vi "HFRR ADV v033 new software.vi"() -> ()   [LabVIEW 2025] (continued)
  # "System Control Commands\nS;1 - Starts the full automation cycle (Runs Priming-humidify till 70RH sequence first, then switches to Maintenance).\nS;0 - Stops the system immediately and enters Standby mode (Safe State: All actuators OFF).\nM;1 - Skips the priming sequence and jumps directly to Maintenance mode (PID control).\nR;1 - Resets the logic state machine and clears all errors, returning to Standby.\nService Mode (Manual Control)\nX;1 - Enters Manual Service Mode. This disables all automatic logic, sensor safety checks, and timers.\nX;0 - Exits Manual Service Mode and returns to Standby (Safe State).\nActuator Commands (Only work after sending X;1)\nP;[0-255] - Sets the Pump PWM. Note that this is Active Low (0 = Max Flow, 255 = Pump OFF).\nF;I;[0-255] - Sets the Intake Fan speed (0 = OFF, 255 = Max Speed).\nF;O;[0-255] - Sets the Exhaust Fan speed (0 = OFF, 255 = Max Speed).\nD;1 - Turns the Dehumidifier Relay ON.\nD;0 - Turns the Dehumidifier Relay OFF."
  # "%RH"
  # "ISO : WS1.4"
  # "Start test and end test log--- done\nDisable heater ON and Humidity ON during the test --- done\ntemprature and ---done\nhumidity reach log\nauto start run true logic and log\nmanual start log once"
  # "Reference Fluid Information"
  # "Note:\nMake sure to place all images in the folder \"C:\\WinDucom\\im\" before clicking on \"Import Image.\""
  # "NOTE:\nPlace all the images in the path \"C:\\WinDucom\\im\" before clicking on Import Image"
  # "Wear Scar Measurements"
  # "Reference Fluid Information"
  # "Graph :"
types:
  T1 = enum32{"Home", "Dashboard", "Imaging", "Report", "Analysis", "About", "Test Setup", "Advance", "Calibration"}
  T2 = enum32{"HOME", "Test Setup", "Acquire", "Adv Scar", "Adv Scar Report", "Compare Files", "Calibration", "About", "Advance", "Mooha"}
  T3 = enum16{"ASTM D6079", "ISO 12156", "CEC F-096-A-06", "Custom"}
  T4 = enum32{"Dashboard 1", "Dashboard 2", "Dashboard 3"}
  T5 = enum32{"COF", "Friction", "ECR", "Temperature", "Humidity", "Stroke"}
  T6 = enum32{"Coefficient Of Friction", "Air Temperature", "Humidity", "Stroke", "Sample Temperature", "Electrical Contact Resistance", "Frequency", "Air Temp vs Rh"}
  T7 = enum32{"Main", "Stroke", "Friction", "Temperature"}
  T8 = enum32{"Stroke Calibration", "Friction Force Calibration", "Temperature Calibration", "Default"}
  T9 = enum32{"Step 1", "Step 2", "Step 3", "Step 4", "Step 5", "Step 6", "Step 7", "Step 8", "Step 9"}
  T10 = enum32{"Test Progress", "Stroke Points Completed"}
  T11 = enum32{"Page 1", "Page 2", "Page 3", "Page 4", "Page 5", "Page 6"}
  T12 = enum32{"Main", "Step 1", "Step 2", "Step 3", "Air Step 1", "Air Step 2", "Air Step 3"}
  T13 = enum32{"Air Temperature", "Sample Temperature", "Default"}
  T14 = enum32{"COMMUNICATION", "CALIBRATION", "Temp Variables", "Camera", "WO 2465 (1)", "WO 2465 (2)", "WO 2465 (3)"}
  T15 = typedef "Auto Start enum.ctl" = enum16{"Init", "Humidity & Temperature On", "Reach point", "Maintain Stage", "Start Stage", "close", "Exit"}
  T16 = typedef "imagedata.ctl" = cluster{"image type":i32, "image depth":i32, "image":u8[], "mask":u8[], "colors":u32[], "Rectangle":cluster{"left":i16, "top":i16, "right":i16, "bottom":i16}}
  T17 = enum32{"HOME", "Test Setup", "Acquire", "Compare Files", "Print Report", "About", "Advance", "Mooha"}
  T18 = cluster{"Read Heave and Surge":string, "Bytes at Heave Port":dbl, "Heave and Surge COM Port:":refnum<visa-resource-name>, "Com Port 2":refnum<visa-resource-name>, "Residual Due":string, "Heave COM Status 2":bool, "Heave COM Status":bool, "Port 2":bool, "Sway PPR":dbl, "Surge PPR":dbl, "Heave PPR":dbl, "Sway Pitch":dbl, "Surge Pitch":dbl, "Heave Pitch":dbl, "Sway Pulses/mm":dbl, "Surge Pulses/mm":dbl, "Heave Pulses/mm":dbl, "inner loop":dbl, "Read Heave and Surge 2":string, "String 36":string, "Write S":bool, "WriteCC1":string[], "Heave COM Loop":i32, "LastCom":string, "EXIT":bool, "Error Heave":errorcluster}
  T19 = enum8{"Enabled", "Disabled", "Disabled and Grayed Out"}
  T20 = cluster{"Read Uno":string, "Bytes at Heave Port":dbl, "UNO COM Port:":refnum<visa-resource-name>, "UNO COM Port: 2":refnum<visa-resource-name>, "Residual Due":string, "UNO COM Status 2":bool, "UNO COM Status":bool, "Port 2":bool, "Sway PPR":dbl, "Surge PPR":dbl, "Heave PPR":dbl, "Sway Pitch":dbl, "Surge Pitch":dbl, "Heave Pitch":dbl, "Sway Pulses/mm":dbl, "Surge Pulses/mm":dbl, "Heave Pulses/mm":dbl, "inner loop":dbl, "Read Heave and Surge 2":string, "String 36":string, "Write S":bool, "WriteCC1":string[], "Heave COM Loop":i32, "LastCom":string, "EXIT":bool, "Error Heave":errorcluster}
  T21 = enum32{"HOME", "Test Setup", "Acquire", "Adv Scar", "Adv Scar Report", "Compare Files", "About", "Advance", "Mooha"}
  T22 = typedef "POST ANALYSIS ENUM.ctl" = enum16{"OPEN EXE", "INIT", "OPEN FILE", "FIT", "DRAW REC", "DRAW LINE", "PAN", "ZOOM IN", "ZOOM OUT", "SET ZOOM", "CLEAR ROI", "GET MEASUREMENTS", "RESIZE MODE", "STREAM START", "STREAM STOP", "SHOW UI", "MINIMIZE UI", "HIDE UI", "CKISE APP", "CLOSE CONNECTION", "SAVE IMAGE", "SET ROI COLOR", "READ", "TCP CHECK", "CLOSE"}
  T23 = typedef "CAMERA LIVE FEED ENUM.ctl" = enum16{"OPEN EXE", "INIT", "READ", "CAMERA CONNECT", "CAMERA START", "CAMERA STOP", "CAMERA GRAY", "CAMERA RGB", "CAMERA MINIMIZE", "CAMERA CLOSE", "CAMERA MODE LIST", "CAMERA MODE SET", "CAMERA RESTORE", "CAMERA SAVE", "CLOSE"}
  T24 = enum16{"Always On", "Always Off", "Off While Running"}
  T25 = enum32{"Home", "Dashboard", "Imaging", "Report", "Analysis", "About", "Test Setup", "Advance"}
  T26 = cluster{"File Name":string, "Test Method":string, "Operator":string, "Fuel Description":string, "Date and time":string}
  T27 = enum32{"Home", "Dashboard", "Imaging", "Report", "Analysis", "About", "Test Setup"}
  T28 = enum32{"HOME", "Test Setup", "Acquire", "Compare Files", "About", "Advance", "Mooha"}
  T29 = typedef "NI_ReportGenerationCore.lvlib/HTML Report Image Alignment.ctl" = enum16{"(default)", "LEFT", "RIGHT", "TOP", "TEXTTOP", "MIDDLE", "ABSMIDDLE", "BASELINE", "BOTTOM", "ABSBOTTOM"}
  T30 = cluster{"y":dbl, "LVDT STROKE DISPLAY":dbl, "y":dbl}
  T31 = enum16{"INIT", "READ", "MANUAL WRITE", "WRITE", "CLOSE", "ERROR INIT"}
diagram:
  w3 = 0.0 ("ch0_filt")
  w5 = -9999999.0 ("max_ch0")
  w6 = 9999999.0 ("min_ch0")
  w17 = FALSE ("Visible")
  w18 = T19."Enabled" ("Disabled")
  w21 = FALSE ("Visible")
  w20 = FALSE ("Humidity Off Command")
  w36 = "" ("USER ID")
  (unwired) T21."HOME" ("Main Tab")
  # "[CH1]    - FF\n[CH2]   - TEMPERATURE\n[CH3]    - Humidity\n[CH4]    - AIR TEMP\n[CH5]\\- Visa Uno\n[CH6] \\- Visa Due\n[CH7]  \\- file path\n[CH8]   - Displacement Gain\n[CHA]   - Stroke Gain\n[CHB]   - Stroke PID Gain\n[CHC]   -Language Selection\n[CHD]   -Power +\n[CHE]   -Power_\n[CHF]   -Heater\n[CHG]   -Humidity Wet\n[CHH]   -Humidity Dry\n[CHI]   -Integral Time \n[CHIJ   -Air intercept\n[CHI]   -Temp Intercept"
  n1 = local write "Cal Password"("" ("Cal Password")) -> ()
  n2 = property on="Auto Start Test" class="Bool (strict)"("Visible"=TRUE) -> ()  [unwired: 2 in, 2 out]
  n3 = property on="FRICVALZ 2" class="Bool (strict)"("DisabledEnum"=w18) -> ()  [unwired: 2 in, 2 out]
  n4 = property on="FRICVALZ 4" class="Bool (strict)"("DisabledEnum"=w18) -> ()  [unwired: 2 in, 2 out]
  n5 = property on="FRICVALZ 3" class="Bool (strict)"("DisabledEnum"=w18) -> ()  [unwired: 2 in, 2 out]
  n6 = property on="About" class="Clust (strict)"("Visible"=FALSE) -> ()  [unwired: 2 in, 2 out]
  n7 = property on="Wrong Password" class="Str"("Visible"=w17) -> ()  [unwired: 2 in, 2 out]
  n8 = property on="Calibration 2" class="TabCtl (strict)"("Visible"=w17) -> ()  [unwired: 2 in, 2 out]
  n9 = flat-sequence {
    tunnel: [w57] -> w2
    tunnel: [w102] -> w28
    tunnel: w2 -> [w97]
    tunnel: [w103] -> w30
    tunnel: w28 -> [w103]
    tunnel: w30 -> [w163]
    tunnel: [w163] -> w29
    tunnel: w29 -> [w194]
    tunnel: [w194] -> w39
    tunnel: w39 -> [w201]
    tunnel: [w207] -> w27
    tunnel: [w195] -> w26
    tunnel: [w249] -> w1
    tunnel: [w248] -> _
    tunnel: w27 -> [w248]
    tunnel: w26 -> [w249]
    frame #0 {
      n10 = call "CLOSE CONNECTION.vi"("error in (no error)"="error in (no error) 2") -> ("error out"=w62:errorcluster)  [unwired: 10 in]
      n11 = call <vilib>:"Clear Errors.vi"("error in (no error)"=w62) -> ("error out"=w61:errorcluster)  [unwired: 5 in, 1 out]
      n12 = disable-structure shown="Enabled" {
        disable-tunnel: w61 -> [w89 _]
        disable-tunnel: [w88 _] -> w60
        frame Enabled {
          n13 = call <userlib>:"Fit VI window to Largest Dec.vi"("error in (no error)"=w89, "border spacing (2 px)"=1) -> ("error out"=w92:errorcluster, "dup VI Ref"=w96:refnum<vi>)  [unwired: 4 in]
          n14 = invoke on="Invoke Node" class="VI" method="FP.Run-Time Position.Maximized"(reference=w96, error in=w92) -> (error out=w93:errorcluster)  [unwired: 2 in, 3 out]
          n15 = call <vilib>:"Clear Errors.vi"("error in (no error)"=w93) -> ("error out"=w95:errorcluster)  [unwired: 5 in, 1 out]
          n16 = control-ref of="This VI"() -> (w87:refnum<vi>)
          n17 = invoke on="Invoke Node" class="VI" method="Default Vals.Reinit All"(reference=w87, error in=w95) -> (reference out=w91:refnum<vi>, error out=w90:errorcluster)  [unwired: 1 in, 1 out]
          n18 = Close Reference(reference=w91, error in (no error)=w90) -> (error out=w88:errorcluster)
        }
        frame Disabled {
        }
      }
      n19 = call "Stall Data Flow.vim"("value in"=w60, "milliseconds to wait"=u32 2000) -> ("value out"=w59:errorcluster)  [unwired: 1 out]
      n20 = call "Read Config.vi"("error in (no error)"=w59) -> ("error out"=w57:errorcluster, "STROKE PARAMETERS"=w68:dbl[], "ADC PARAMETERS"=w69:dbl[], "PID  PARAMETERS"=w70:dbl[], "Stroke Calibration"=w67:string)  [unwired: 6 in]
      n21 = Index Array(array=w68) -> (element #1=w85:dbl, element #2=w86:dbl)  [unwired: 2 in]
      n22 = Index Array(array=w69) -> (element #1=w81:dbl, element #2=w82:dbl, element #3=w83:dbl, element #4=w84:dbl)  [unwired: 4 in]
      n23 = Index Array(array=w70) -> (element #1=w72:dbl, element #2=w73:dbl, element #3=w74:dbl, element #4=w75:dbl, element #5=w76:dbl, element #6=w77:dbl, element #7=w78:dbl, element #8=w79:dbl, element #9=w80:dbl)  [unwired: 9 in]
      n24 = local write "milliseconds to wait"(w72) -> ()
      n25 = local write "dt"(w73) -> ()
      n26 = local write "kp"(w74) -> ()
      n27 = local write "ki"(w75) -> ()
      n28 = local write "kd"(w76) -> ()
      n29 = local write "max_step_change"(w77) -> ()
      n30 = local write "max_amplitude"(w78) -> ()
      n31 = local write "min_amplitude"(w79) -> ()
      n32 = local write "startup_cmd"(w80) -> ()
      n33 = local write "VREF"(w81) -> ()
      n34 = local write "ADC_Resolution"(w82) -> ()
      n35 = local write "PIEZO_CAL_FACTOR"(w83) -> ()
      n36 = local write "NORMAL_FORCE"(w84) -> ()
      n37 = local write "STROKE FILTER"(w85) -> ()
      n38 = local write "Add up Stroke"(w86) -> ()
      n39 = Spreadsheet String To Array(delimiter (Tab)=";", format string="", spreadsheet string=w67, array type (2D Dbl)=dbl[] []) -> (array=w71:dbl[])
      n40 = local write "calibration values"(w71) -> ()
    }
    frame #1 {
      n41 = property on="Auto Scar Check" class="Clust (strict)"("Visible"=TRUE) -> ()  [unwired: 2 in, 2 out]
      n42 = property on="Sign In" class="Bool (strict)"("DisabledEnum"=T19."Disabled" ("Disabled")) -> ()  [unwired: 2 in, 2 out]
      n43 = local write "sign in temp"(FALSE ("sign in temp")) -> ()
      n44 = call "dialog box.vi"("Status"="Before starting the test, verify that the microscope cable is connected.", "error in"=w97) -> ("error out"=w102:errorcluster)  [unwired: 8 in]
    }
    frame #2 {
      (unwired) TRUE ("Re-Initialise")
      # "kkkkk"
      # "C:\\Windows\\wndcm_pw_stdED hfrr.txt"
      # "C:\\LAB-IQ NXT"
      # "C:\\LAB-IQ NXT\\wndcm_pw_stdED hfrr.txt"
      # "password file"
      n45 = Current VI's Path() -> (path=w119:path)
      n46 = Strip Path(path=w119) -> (stripped path=w112:path)  [unwired: 1 out]
      n47 = local write "main tab sub"(enum32{"Page 1", "Page 2"}."Page 1" ("main tab sub")) -> ()
      n48 = local write "Main Tab Display"(T4."Dashboard 1" ("Main Tab Display")) -> ()
      n49 = local write "Main Tab"(T2."HOME" ("Main Tab")) -> ()
      n50 = Path To String(path=w112) -> (string=w114:string)
      n51 = Search/Split String(string=w114, search string/char (-)=".exe") -> (match + rest of string=w116:string)  [unwired: 1 in, 2 out]
      n52 = Match True/False String(2:".vi" ("false string"), 3:".exe" ("true string"), 4:w116) -> (0:w113:bool)  [unwired: 1 out]
      n53 = List Folder(path=path "C:/LAB-IQ" ("directory path"), pattern="*.txt") -> (filenames=w125:string[])  [unwired: 2 in, 3 out]
      n54 = case shown="True" w113 {
        tunnel: w112 -> [w134 w136]
        tunnel: [w134 w135] -> w110
        frame False {
        }
        frame True {
          n55 = Strip Path(path=w136) -> (stripped path=w135:path)  [unwired: 1 out]
        }
      }
      n56 = Search 1D Array(1D array=w125, element="wndcm_pw_stdED hfrr.txt") -> (index of element=w128:i32)  [unwired: 1 in]
      n57 = Equal?(x=w128, y=-1) -> (x = y?=w123:bool)
      n58 = Path To String(path=w110) -> (string=→"Gain path":string)
      n59 = case shown="True" w123 {
        frame False {
        }
        frame True {
          n60 = String To Byte Array(string="123\n") -> (unsigned byte array=w141:u8[])
          n61 = Array Size(array=w141) -> (size(s)=w140:i32)
          n62 = for {
            N: w140 -> [_]
            tunnel: w141 -> [w154]
            tunnel: [w151] -> w143 mode=indexing
            tunnel: w140 -> [w146]
            i -> [w144]
            n63 = Decrement(x=w146) -> (x-1=w147:i32)
            n64 = Index Array(array=w154, index=w144) -> (element=w153:u8)
            n65 = Equal?(x=w144, y=w147) -> (x = y?=w148:bool)
            n66 = Number To Decimal String(number=w153) -> (decimal integer string=w152:string)  [unwired: 1 in]
            n67 = Select(t="", s=w148, f="\r") -> (s? t:f=w145:string)
            n68 = Concatenate Strings(w152, w145) -> (w151:string)
          }
          n69 = local read "file path"() -> (w137:path)
          n70 = Concatenate Strings(w143) -> (w139:string)
          n71 = call <vilib>:"Write Characters To File.vi"("append to file? (new file:F)"=FALSE, "character string"=w139, "file path (dialog if empty)"=w137) -> ()  [unwired: 2 in, 1 out]
        }
      }
      n72 = local write "conststatus"(0.0 ("rpm value : 2")) -> ()
      n73 = local write "EVENT LOG"("") -> ()
      n74 = local write "COUNT"(0 ("COUNT")) -> ()
      n75 = local write "clk"(0.0 ("clk")) -> ()
      n76 = local write "Flag"(0.0 ("Flag")) -> ()
      n77 = local write "Lan flag"(0.0 ("Lan flag")) -> ()
      n78 = local write "Com flag"(u32 0 ("Com flag")) -> ()
      n79 = local write "refresh flag"(FALSE ("refresh flag")) -> ()
      "file path" <- path "C:/LAB-IQ/wndcm_pw_stdED hfrr.txt" ("file path")
      "FF buffer" <- dbl[] [] ("FF buffer")
    }
    frame #3 {
      # "C:\\WinDucom\\calibrate WO 2391.dcf"
      n80 = String To Path(string="C:\\LAB-IQ\\Image Calibrate v01.dcf") -> (path=w158:path)
      n81 = String To Path(string="C:\\LAB-IQ\\calibrate WO 2465.dcf") -> (path=w162:path)
      n82 = Open/Create/Replace File "Open File"(file path (use dialog)=w162) -> (refnum out=w161:refnum<file>)  [unwired: 5 in, 2 out]
      n83 = Open/Create/Replace File ("Open File")(file path (use dialog)=w158) -> (refnum out=w157:refnum<file>)  [unwired: 5 in, 2 out]
      n84 = for {
        N: 4 -> [_]
        tunnel: w157 -> [w169]
        i -> [w165]
        n85 = Read from Text File ("Read File")(file (use dialog)=w169) -> (text=w170:string)  [unwired: 3 in, 3 out]
        n86 = String Subset(string=w170, offset (0)=6, length (rest)=10 ("length (rest)")) -> (substring=w166:string)
        n87 = Fract/Exp String To Number(string=w166) -> (number=w164:dbl)  [unwired: 3 in, 1 out]
        n88 = case shown="3" w165 {
          tunnel: w164 -> [w171 w172 _ w173 _]
          frame 0 {
            n89 = local write "5x Gain"(w171) -> ()
          }
          frame 1 {
            n90 = local write "10x Gain"(w172) -> ()
          }
          frame 2 {
          }
          frame 3 {
            n91 = local write "100x gain"(w173) -> ()
          }
          frame 4, Default {
          }
        }
      }
      n92 = for {
        N: 24 -> [_]
        tunnel: w161 -> [w182]
        i -> [w176]
        (unwired) TRUE ("line mode (F)")
        n93 = Read from Text File "Read File"(file (use dialog)=w182) -> (text=w181:string)  [unwired: 3 in, 3 out]
        n94 = Match Pattern(string=w181, regular expression="]") -> (after substring=w179:string)  [unwired: 1 in, 3 out]
        n95 = String Subset(string=w181, offset (0)=5, length (rest)=10 ("length (rest)")) -> (substring=w174:string)
        n96 = Fract/Exp String To Number(string=w174) -> (number=w175:dbl)  [unwired: 3 in, 1 out]
        n97 = Match Pattern(string=w179, regular expression="-") -> (before substring=w177:string)  [unwired: 1 in, 3 out]
        n98 = case shown="18" w176 {
          tunnel: w175 -> [_ _ _ _ _ _ _ _ _ _ w189 _ _ _ _ _ _ _ _ _ _ _ _ _ _]
          tunnel: w177 -> [_ _ _ _ w185 w186 w187 _ _ _ _ _ _ _ _ _ _ _ _ _ w190 _ w191 w192 _]
          frame 0 {
          }
          frame 1 {
          }
          frame 2 {
          }
          frame 3 {
          }
          frame 4 {
            n99 = local write "Com Port 1"(w185) -> ()
          }
          frame 5 {
            n100 = local write "Com Port 2"(w186) -> ()
            n101 = local write "visa due"(w186) -> ()
          }
          frame 6 {
            n102 = String To Path(string=w187) -> (path=w188:path)
            n103 = local write "File Path"(w188) -> ()
          }
          frame 7 {
          }
          frame 8 {
          }
          frame 9 {
          }
          frame 10 {
            n104 = local write "Language Selection"(w189) -> ()
          }
          frame 11 {
          }
          frame 12 {
          }
          frame 13 {
          }
          frame 14 {
          }
          frame 15 {
          }
          frame 16 {
          }
          frame 17 {
          }
          frame 18 {
          }
          frame 21 {
          }
          frame 22 {
            n105 = local write "Com Port 3"(w190) -> ()
          }
          frame 23 {
          }
          frame 19 {
            n106 = local write "C3 :"(w191) -> ()
          }
          frame 20 {
            n107 = local write "Camera Port :"(w192) -> ()
          }
          frame 24, Default {
          }
        }
      }
    }
    frame #4 {
      n108 = Wait (ms)(milliseconds to wait=u32 1000) -> ()  [unwired: 1 out]
    }
    frame #5 {
      w210 = u32 2000 ("milliseconds to wait")
      w237 = u32 2000 ("milliseconds to wait")
      n109 = call "CAMERA LIVE FEED FGV.vi"("Enum - Menu"=CAMERA_LIVE_FEED_ENUM."OPEN EXE", "error in (no error)"=w201) -> ("error out"=w243:errorcluster)  [unwired: 8 in, 1 out]
      n110 = call "IMAGE ANALYSIS.vi"("Enum"=POST_ANALYSIS_ENUM."OPEN EXE", "error in"=w201) -> ("error out"=w198:errorcluster)  [unwired: 8 in, 1 out]
      n111 = call "Stall Data Flow.vim"("value in"=w243, "milliseconds to wait"=w237) -> ("value out"=w241:errorcluster)  [unwired: 1 out]
      n112 = call "Stall Data Flow.vim"("value in"=w198, "milliseconds to wait"=u32 8000) -> ("value out"=w197:errorcluster)  [unwired: 1 out]
      n113 = call "CAMERA LIVE FEED FGV.vi"("Enum - Menu"=CAMERA_LIVE_FEED_ENUM."INIT", "error in (no error)"=w241) -> ("error out"=w239:errorcluster)  [unwired: 8 in, 1 out]
      n114 = call "IMAGE ANALYSIS.vi"("Enum"=POST_ANALYSIS_ENUM."INIT", "error in"=w197) -> ("error out"=w195:errorcluster)  [unwired: 8 in, 1 out]
      n115 = case shown="Error .." w239 {
        selector: w239 -> [w244 _]
        tunnel: [w244 _] -> w238
        frame No Error {
        }
        frame Error {
          n116 = One Button Dialog(message="Camera initialization error.\nPlease Restart the software") -> ()  [unwired: 1 in, 1 out]
        }
      }
      n117 = property on="Camera Port :" class="CmbBox"() -> ("Strings[]"=w235:string[], "Value"=w236:string)  [unwired: 2 in, 2 out]
      n118 = Search 1D Array(1D array=w235, element=w236) -> (index of element=w234:i32)  [unwired: 1 in]
      n119 = Type Cast(type=30, x=w234) -> (*(type *) &x=w232:i32)
      n120 = call "Stall Data Flow.vim"("value in"=w238, "milliseconds to wait"=w237) -> ("value out"=w214:errorcluster)  [unwired: 1 out]
      n121 = Add(x=w232, y=48) -> (x+y=w213:i32)
      n122 = call "CAMERA LIVE FEED FGV.vi"("Enum - Menu"=CAMERA_LIVE_FEED_ENUM."CAMERA CONNECT", "error in (no error)"=w214, "CAMERA PORT"=w213) -> ("error out"=w223:errorcluster)  [unwired: 7 in, 1 out]
      n123 = call "Stall Data Flow.vim"("value in"=w223, "milliseconds to wait"=u32 5000) -> ("value out"=w224:errorcluster)  [unwired: 1 out]
      n124 = call "CAMERA LIVE FEED FGV.vi"("Enum - Menu"=CAMERA_LIVE_FEED_ENUM."CAMERA MODE LIST", "error in (no error)"=w224) -> ("error out"=w226:errorcluster)  [unwired: 8 in, 1 out]
      n125 = call "Stall Data Flow.vim"("value in"=w226, "milliseconds to wait"=w210) -> ("value out"=w225:errorcluster)  [unwired: 1 out]
      n126 = call "CAMERA LIVE FEED FGV.vi"("Enum - Menu"=CAMERA_LIVE_FEED_ENUM."READ", "error in (no error)"=w225) -> ("error out"=w212:errorcluster, "data out"=→"Camera List":string)  [unwired: 8 in]
      n127 = Type Cast(type=30, x=0) -> (*(type *) &x=w206:i32)
      n128 = call "Stall Data Flow.vim"("value in"=w212, "milliseconds to wait"=w210) -> ("value out"=w211:errorcluster)  [unwired: 1 out]
      n129 = Add(x=w206, y=48) -> (x+y=w204:i32)
      n130 = call "CAMERA LIVE FEED FGV.vi"("Enum - Menu"=CAMERA_LIVE_FEED_ENUM."CAMERA MODE SET", "error in (no error)"=w211, "CAMERA MODE"=w204) -> ("error out"=w208:errorcluster)  [unwired: 7 in, 1 out]
      n131 = call "Stall Data Flow.vim"("value in"=w208, "milliseconds to wait"=u32 2000) -> ("value out"=w228:errorcluster)  [unwired: 1 out]
      n132 = call "CAMERA LIVE FEED FGV.vi"("Enum - Menu"=CAMERA_LIVE_FEED_ENUM."CAMERA START", "error in (no error)"=w228) -> ("error out"=w229:errorcluster)  [unwired: 8 in, 1 out]
      n133 = call "Stall Data Flow.vim"("value in"=w229, "milliseconds to wait"=u32 1000) -> ("value out"=w230:errorcluster)  [unwired: 1 out]
      n134 = call "CAMERA LIVE FEED FGV.vi"("Enum - Menu"=CAMERA_LIVE_FEED_ENUM."CAMERA MINIMIZE", "error in (no error)"=w230) -> ("error out"=w207:errorcluster)  [unwired: 8 in, 1 out]
    }
    frame #6 {
      n135 = case shown="No Error" w248 {
        frame No Error {
          n136 = property on="Auto Scar Check" class="Clust (strict)"("Visible"=FALSE) -> ()  [unwired: 2 in, 2 out]
        }
        frame Error {
        }
      }
      n137 = property on="Sign In" class="Bool (strict)"("DisabledEnum"=T19."Enabled" ("Disabled")) -> ()  [unwired: 2 in, 2 out]
      n138 = local write "sign in temp"(TRUE ("sign in temp")) -> ()
    }
  }
  n139 = local write "SCAR MEASURMENT"(enum32{"Auto Scar", "Manual Scar"}."Manual Scar" ("SCAR MEASURMENT")) -> ()
  n140 = local write "Temperature Off Command"(w20) -> ()
  n141 = local write "Main Dashboard Buttons"(T1."Home" ("Main Dashboard Buttons")) -> ()
  n142 = local write "Humidity Off Command"(w20) -> ()
  n143 = local write "CAMERA ROI MIN TEMP"(w20) -> ()
  n144 = local write "TEST FILE NAM,E SAVED"(w20) -> ()
  n145 = local write "LIVE FEED MIN TEMP"(w20) -> ()
  n146 = local write "SCAR MEASURMENT"(enum32{"Auto Scar", "Manual Scar"}."Manual Scar" ("SCAR MEASURMENT")) -> ()
  n147 = local write "Auto stop temp"(w21) -> ()
  n148 = local write "main tab sub"(enum32{"Page 1", "Page 2"}."Page 1" ("main tab sub")) -> ()
  n149 = local write "USERNAME"(w36) -> ()
  n150 = local write "Main Tab"(T2."HOME" ("Main Tab")) -> ()
  n151 = local write "USER ID"(w36) -> ()
  n152 = property on="Auto Scar Check  2" class="Clust (strict)"("Visible"=w21) -> (error out=w24:errorcluster)  [unwired: 2 in, 1 out]
  n153 = property on="Quit" class="Bool (strict)"("Value"=FALSE ("Quit")) -> (error out=w38:errorcluster)  [unwired: 2 in, 1 out]
  n154 = while {
    stop <- w251 stop-if-true
    n155 = event shown="[7] \"Heater Button\": Value Change" {
      selector: _ -> [_ _ _ _ _ _ _ _ _ _ _ _ _ _ _ _ _ _ _ _ _ _ _ _ _ _ _ _ _ _ _ _ _ _ _ _ _ _ _ _ _ _ _ _ _ _ _ _ _]
      dyn-events: _ -> [_ _ _ _ _ _ _ _ _ _ _ _ _ _ _ _ _ _ _ _ _ _ _ _ _ _ _ _ _ _ _ _ _ _ _ _ _ _ _ _ _ _ _ _ _ _ _ _ _]
      timeout: 100 -> [_ _ _ _ _ _ _ _ _ _ _ _ _ _ _ _ _ _ _ _ _ _ _ _ _ _ _ _ _ _ _ _ _ _ _ _ _ _ _ _ _ _ _ _ _ _ _ _ _]
      tunnel: [FALSE FALSE FALSE _ FALSE _ _ _ _ _ _ _ _ _ _ _ _ _ _ _ _ _ _ _ _ _ _ _ _ _ _ _ _ _ _ _ _ _ _ _ _ _ _ _ _ _ _ _ TRUE] -> w251
      event Timeout {
        n156 = event-data() -> ()  [unwired: 1 in, 3 out]
        n157 = disable-structure shown="Disabled" {
          frame Disabled {
            n158 = local read "Auto Start Test"() -> (w265:bool)
            n159 = local read "RUN"() -> (w266:bool)
            n160 = Or(x=w266, y=w265) -> (x .or. y?=w264:bool)
            n161 = case shown="True" w264 {
              frame False {
                w267 = TRUE ("PAUSE")
                n162 = call "ELAPSED TIMER VI - abort test.vi"("RESET"=w267, "PAUSE"=w267) -> ()  [unwired: 7 in, 3 out]
              }
              frame True {
                n163 = local read "Stroke 2"() -> (w272:dbl)
                n164 = local read "FF 3"() -> (w274:dbl)
                n165 = Equal?(x=w272, y=0.95 ("Stroke 2")) -> (x = y?=w269:bool)
                n166 = Equal?(x=w274, y=0.0 ("FF 3")) -> (x = y?=w270:bool)
                n167 = Or(x=w270, y=w269) -> (x .or. y?=w268:bool)
                n168 = case shown="True" w268 {
                  selector: w268 -> [_ w279]
                  frame False {
                    w275 = TRUE ("PAUSE")
                    n169 = call "ELAPSED TIMER VI - abort test.vi"("RESET"=w275, "PAUSE"=w275) -> ()  [unwired: 7 in, 3 out]
                  }
                  frame True {
                    n170 = Not(x=w279) -> (.not. x?=w278:bool)
                    n171 = call "ELAPSED TIMER VI - abort test.vi"("TARGET"=60.0, "RESET"=w278, "PAUSE"=FALSE) -> ("ELAPSED INDICATION"=w276:bool)  [unwired: 6 in, 2 out]
                    n172 = case shown="True" w276 {
                      frame False {
                      }
                      frame True {
                        n173 = stacked-sequence {
                          frame #0 {
                            w281 = FALSE
                            n174 = local write "RUN"(w281) -> ()
                            n175 = local write "Auto Start Test"(w281) -> ()
                          }
                          frame #1 {
                            n176 = One Button Dialog(message="Test stopped due to a communication error. Reconnect the C1 and C2 cables.") -> ()  [unwired: 1 in, 1 out]
                          }
                        }
                      }
                    }
                  }
                }
              }
            }
          }
          frame Enabled {
          }
        }
        n177 = Get Date/Time In Seconds() -> (seconds since 1Jan1904=w262:timestamp)
        n178 = Format Into String(format string="%<%I:%M:%S:%p %d:%B:%Y>T", w262) -> (resulting string=→"Time Stamp":string)  [unwired: 2 in, 1 out]
        n179 = local read "Service Password enable"() -> (w254:bool)
        n180 = local read "FILE"() -> (w259:string)
        n181 = call <vilib>:"Trim Whitespace.vi"("string"=w259) -> ("trimmed string"=w258:string)  [unwired: 1 in]
        n182 = String Length(string=w258) -> (length=w257:i32)
        n183 = Greater?(x=w257, y=1) -> (0:w255:bool)
        n184 = case shown="False" w255 {
          tunnel: w254 -> [w283 _]
          frame False {
            n185 = case shown="False" w283 {
              frame True {
                w284 = "Test Start In Service Mode" ("Tip Strip")
                w285 = T19."Enabled" ("Disabled")
                n186 = property on="Auto Start Test" class="Bool (strict)"("DisabledEnum"=w285, "TipStrip"=w284) -> ()  [unwired: 2 in, 2 out]
                n187 = property on="RUN" class="Bool (strict)"("DisabledEnum"=w285, "TipStrip"=w284) -> ()  [unwired: 2 in, 2 out]
              }
              frame False {
                w286 = "Enter File Name to Start Test" ("Tip Strip")
                w287 = T19."Disabled and Grayed Out" ("Disabled")
                n188 = property on="Auto Start Test" class="Bool (strict)"("DisabledEnum"=w287, "TipStrip"=w286) -> ()  [unwired: 2 in, 2 out]
                n189 = property on="RUN" class="Bool (strict)"("DisabledEnum"=w287, "TipStrip"=w286) -> ()  [unwired: 2 in, 2 out]
              }
            }
          }
          frame True {
            w288 = "" ("Tip Strip")
            w289 = T19."Enabled" ("Disabled")
            n190 = property on="Auto Start Test" class="Bool (strict)"("DisabledEnum"=w289, "TipStrip"=w288) -> ()  [unwired: 2 in, 2 out]
            n191 = property on="RUN" class="Bool (strict)"("DisabledEnum"=w289, "TipStrip"=w288) -> ()  [unwired: 2 in, 2 out]
          }
        }
      }
      event "RUN": Value Change {
        n192 = event-data() -> ()  [unwired: 1 in, 6 out]
        n193 = local read "RUN"() -> (w291:bool)
        n194 = case shown="True" w291 {
          frame False {
            n195 = flat-sequence {
              frame #0 {
                n196 = local write "START TEMP"(FALSE ("START TEMP")) -> ()
              }
              frame #1 {
                n197 = Wait (ms)(milliseconds to wait=u32 1500) -> ()  [unwired: 1 out]
              }
              frame #2 {
              }
              frame #3 {
                n198 = local write "Due Write"("VC;0") -> ()
              }
              frame #4 {
                n199 = Wait (ms)(milliseconds to wait=u32 1500) -> ()  [unwired: 1 out]
              }
              frame #5 {
                w300 = T19."Enabled" ("Disabled")
                (unwired) T25."Imaging" ("Main Dashboard Buttons")
                (unwired) T21."Adv Scar" ("Main Tab")
                w302 = "" ("FILE")
                n200 = local write "measured_stroke"(0.0 ("measured_stroke")) -> ()
                n201 = local write "Due Write"("VC;0") -> ()
                n202 = local write "FILE"(w302) -> ()
                n203 = local write "Batch Ref Num :"(w302) -> ()
                n204 = local write "Fuel Discription :"(w302) -> ()
                n205 = local write "Main Tab"(T2."Adv Scar" ("Main Tab")) -> ()
                n206 = local write "Remarks :"(w302) -> ()
                n207 = local write "Main Dashboard Buttons"(T1."Imaging" ("Main Dashboard Buttons")) -> ()
                n208 = local write "TEST FILE NAM,E SAVED"(FALSE ("TEST FILE NAM,E SAVED")) -> ()
                n209 = property on="Stroke ( mm )" class="WFChart (strict)"("History Data"=cluster{"y":dbl, dbl, "y":dbl}[] []) -> ()  [unwired: 2 in, 2 out]
                n210 = property on="Auto Start Test" class="Bool (strict)"("Visible"=TRUE) -> ()  [unwired: 2 in, 2 out]
                n211 = property on="FRICVALZ 2" class="Bool (strict)"("DisabledEnum"=w300) -> ()  [unwired: 2 in, 2 out]
                n212 = property on="FRICVALZ 4" class="Bool (strict)"("DisabledEnum"=w300) -> ()  [unwired: 2 in, 2 out]
                n213 = property on="FRICVALZ 3" class="Bool (strict)"("DisabledEnum"=w300) -> ()  [unwired: 2 in, 2 out]
              }
            }
          }
          frame True {
            n214 = stacked-sequence {
              frame #0 {
                n215 = local write "Due Write"("DAC;200") -> ()
              }
              frame #1 {
                n216 = Wait (ms)(milliseconds to wait=u32 1500) -> ()  [unwired: 1 out]
              }
              frame #2 {
                n217 = local write "Due Write"("DAC;200") -> ()
              }
              frame #3 {
                n218 = Wait (ms)(milliseconds to wait=u32 1500) -> ()  [unwired: 1 out]
              }
              frame #4 {
                n219 = local write "Due Write"("VC;1") -> ()
              }
              frame #5 {
                n220 = Wait (ms)(milliseconds to wait=u32 2000) -> ()  [unwired: 1 out]
              }
              frame #6 {
                n221 = local write "Due Write"("VC;1") -> ()
              }
              frame #7 {
                n222 = Wait (ms)(milliseconds to wait=u32 2000) -> ()  [unwired: 1 out]
              }
              frame #8 {
                w314 = T19."Disabled" ("Disabled")
                n223 = property on="Auto Start Test" class="Bool (strict)"("Visible"=FALSE) -> ()  [unwired: 2 in, 2 out]
                n224 = local write "START TEMP"(TRUE ("START TEMP")) -> ()
                n225 = property on="FRICVALZ 2" class="Bool (strict)"("DisabledEnum"=w314) -> ()  [unwired: 2 in, 2 out]
                n226 = property on="FRICVALZ 4" class="Bool (strict)"("DisabledEnum"=w314) -> ()  [unwired: 2 in, 2 out]
                n227 = property on="FRICVALZ 3" class="Bool (strict)"("DisabledEnum"=w314) -> ()  [unwired: 2 in, 2 out]
              }
            }
          }
        }
      }
      event "run test Calibration": Value Change {
        n228 = event-data() -> ()  [unwired: 1 in, 6 out]
        n229 = local read "run test Calibration"() -> (w316:bool)
        n230 = case shown="True" w316 {
          frame False {
            n231 = flat-sequence {
              frame #0 {
                n232 = local write "START TEMP"(FALSE ("START TEMP")) -> ()
              }
              frame #1 {
                n233 = Wait (ms)(milliseconds to wait=u32 1500) -> ()  [unwired: 1 out]
              }
              frame #2 {
              }
              frame #3 {
                n234 = local write "Due Write"("VC;0") -> ()
              }
              frame #4 {
                n235 = Wait (ms)(milliseconds to wait=u32 1500) -> ()  [unwired: 1 out]
              }
              frame #5 {
                n236 = local write "Due Write"("VC;0") -> ()
              }
            }
          }
          frame True {
            n237 = flat-sequence {
              frame #0 {
                n238 = local write "Due Write"("VC;1") -> ()
              }
              frame #1 {
                n239 = Wait (ms)(milliseconds to wait=u32 2000) -> ()  [unwired: 1 out]
              }
              frame #2 {
                n240 = local write "Due Write"("VC;1") -> ()
              }
              frame #3 {
                n241 = Wait (ms)(milliseconds to wait=u32 2000) -> ()  [unwired: 1 out]
              }
              frame #4 {
                n242 = local write "START TEMP"(TRUE ("START TEMP")) -> ()
              }
            }
          }
        }
      }
      event "Auto": Value Change {
        n243 = event-data() -> ()  [unwired: 1 in, 6 out]
        n244 = stacked-sequence {
          frame #0 {
            n245 = local write "FILE"("") -> ()
          }
          frame #1 {
            n246 = Get Date/Time In Seconds() -> (seconds since 1Jan1904=w332:timestamp)
            n247 = Format Into String(format string="%<%I_%M_%S_%p_%d_%B_%Y>T", w332) -> (resulting string=w331:string)  [unwired: 2 in, 1 out]
            n248 = local write "FILE"(w331) -> ()
          }
        }
        n249 = local read "Auto"() -> (w329:bool)
        n250 = Not(x=w329) -> (.not. x?=w328:bool)
        n251 = local write "Auto"(w328) -> ()
      }
      event "Auto Start Temp": Value Change {
        n252 = event-data() -> ()  [unwired: 1 in, 6 out]
        n253 = local read "Auto Start Test"() -> (w335:bool)
        n254 = case shown="True" w335 {
          frame False {
            n255 = stacked-sequence {
              frame #0 {
                n256 = local write "START TEMP"(FALSE ("START TEMP")) -> ()
              }
              frame #1 {
                n257 = Wait (ms)(milliseconds to wait=u32 2000) -> ()  [unwired: 1 out]
              }
              frame #2 {
                n258 = local write "Due Write"("VC;0") -> ()
              }
              frame #3 {
                n259 = Wait (ms)(milliseconds to wait=u32 2000) -> ()  [unwired: 1 out]
              }
              frame #4 {
                w345 = T19."Enabled" ("Disabled")
                (unwired) T25."Imaging" ("Main Dashboard Buttons")
                w346 = "" ("FILE")
                n260 = local write "Main Tab"(T2."Adv Scar" ("Main Tab")) -> ()
                n261 = local write "measured_stroke"(0.0 ("measured_stroke")) -> ()
                n262 = local write "Main Dashboard Buttons"(T1."Imaging" ("Main Dashboard Buttons")) -> ()
                n263 = property on="RUN" class="Bool (strict)"("Visible"=TRUE) -> ()  [unwired: 2 in, 2 out]
                n264 = local write "Due Write"("VC;0") -> ()
                n265 = local write "TEST FILE NAM,E SAVED"(FALSE ("TEST FILE NAM,E SAVED")) -> ()
                n266 = local write "Fuel Discription :"(w346) -> ()
                n267 = local write "Batch Ref Num :"(w346) -> ()
                n268 = local write "Remarks :"(w346) -> ()
                n269 = local write "FILE"(w346) -> ()
                n270 = property on="FRICVALZ 2" class="Bool (strict)"("DisabledEnum"=w345) -> ()  [unwired: 2 in, 2 out]
                n271 = property on="FRICVALZ 4" class="Bool (strict)"("DisabledEnum"=w345) -> ()  [unwired: 2 in, 2 out]
                n272 = property on="FRICVALZ 3" class="Bool (strict)"("DisabledEnum"=w345) -> ()  [unwired: 2 in, 2 out]
              }
            }
          }
          frame True {
            n273 = stacked-sequence {
              frame #0 {
                n274 = local write "Due Write"("DAC;200") -> ()
              }
              frame #1 {
                n275 = Wait (ms)(milliseconds to wait=u32 1500) -> ()  [unwired: 1 out]
              }
              frame #2 {
                n276 = local write "Due Write"("DAC;200") -> ()
              }
              frame #3 {
                n277 = Wait (ms)(milliseconds to wait=u32 1000) -> ()  [unwired: 1 out]
              }
              frame #4 {
                n278 = local write "Due Write"("VC;1") -> ()
              }
              frame #5 {
                n279 = Wait (ms)(milliseconds to wait=u32 2000) -> ()  [unwired: 1 out]
              }
              frame #6 {
                n280 = local write "Due Write"("VC;1") -> ()
              }
              frame #7 {
                n281 = Wait (ms)(milliseconds to wait=u32 2000) -> ()  [unwired: 1 out]
              }
              frame #8 {
                w357 = T19."Disabled" ("Disabled")
                n282 = property on="RUN" class="Bool (strict)"("Visible"=FALSE) -> ()  [unwired: 2 in, 2 out]
                n283 = property on="FRICVALZ 2" class="Bool (strict)"("DisabledEnum"=w357) -> ()  [unwired: 2 in, 2 out]
                n284 = property on="FRICVALZ 4" class="Bool (strict)"("DisabledEnum"=w357) -> ()  [unwired: 2 in, 2 out]
                n285 = property on="FRICVALZ 3" class="Bool (strict)"("DisabledEnum"=w357) -> ()  [unwired: 2 in, 2 out]
                "START TEMP" <- TRUE
              }
            }
          }
        }
      }
      event "FILE", "USERNAME", "USER ID": Mouse Enter {
        n286 = event-data() -> ()  [unwired: 1 in, 4 out]
        n287 = dll-call lib="kernel32.dll" fn="Wow64DisableWow64FsRedirection"("OldValue"=0) -> (error out=w364:errorcluster, "OldValue"=w362:i32)  [unwired: 4 in, 1 out]
        n288 = call <vilib>:"System Exec.vi"("run minimized? (F)"=TRUE, "error in (no error)"=w364, "command line"="C:\\Program Files\\Common Files\\Microsoft Shared\\Ink\\TabTip.exe") -> ("error out"=w363:errorcluster)  [unwired: 5 in, 3 out]
        n289 = dll-call lib="kernel32.dll" fn="Wow64EnableWow64FsRedirection"(error in=w363, "OldValue"=w362) -> ()  [unwired: 4 in, 2 out]
      }
      event "EDIT": Value Change {
        n290 = event-data() -> ()  [unwired: 1 in, 6 out]
        n291 = local read "EDIT"() -> (w365:bool)
        n292 = case shown="False" w365 {
          frame False {
            n293 = control-ref of="This VI"() -> (w382:refnum<vi>)
            n294 = property class="VI"(reference=w382) -> (reference out=w373:refnum<vi>, error out=w377:errorcluster, "Panel"=w381:refnum<vi>)  [unwired: 1 in]
            n295 = property class="Pnl"(reference=w381, error in=w377) -> (reference out=w375:refnum<vi>, error out=w378:errorcluster, "Panes[]"=w380:refnum<vi>[])
            n296 = for {
              tunnel: w380 -> [w388] mode=indexing
              tunnel: T24."Always Off" ("Horizontal Scrollbar Visibility") -> [w387]
              tunnel: w378 -> [w384]
              tunnel: [w383] -> w376
              n297 = property class="Pane"(reference=w388, error in=w384, "HorizScrollbarVisibility"=w387) -> (reference out=w385:refnum<vi>, error out=w386:errorcluster)
              n298 = Close Reference(reference=w385, error in (no error)=w386) -> (error out=w383:errorcluster)
            }
            n299 = Close Reference(reference=w375, error in (no error)=w376) -> (error out=w374:errorcluster)
            n300 = Close Reference(reference=w373, error in (no error)=w374) -> (error out=w368:errorcluster)
            "error out 7" <- w368
            n301 = call <vilib>:"Clear Errors.vi"("error in (no error)"=w368) -> ("error out"=w367:errorcluster)  [unwired: 5 in, 1 out]
            n302 = local write "Service Password enable"(FALSE ("Service Password enable")) -> ()
            n303 = call <userlib>:"Fit VI window to Largest Dec.vi"("error in (no error)"=w367, "border spacing (2 px)"=1) -> ("error out"=w372:errorcluster, "dup VI Ref"=w370:refnum<vi>)  [unwired: 4 in]
            n304 = invoke on="Invoke Node" class="VI" method="FP.Run-Time Position.Maximized"(reference=w370, error in=w372) -> (error out=w371:errorcluster)  [unwired: 2 in, 3 out]
            n305 = call <vilib>:"Clear Errors.vi"("error in (no error)"=w371) -> ()  [unwired: 5 in, 2 out]
          }
          frame True {
          }
        }
      }
      event "Heater Button": Value Change {
        n306 = event-data() -> ()  [unwired: 1 in, 6 out]
        n307 = local read "Heater Button"() -> (w389:bool)
        n308 = case shown="True" w389 {
          frame True {
            n309 = stacked-sequence {
              frame #0 {
                n310 = Wait (ms)(milliseconds to wait=u32 1500) -> ()  [unwired: 1 out]
              }
              frame #1 {
                n311 = local read "Set Temp"() -> (w391:dbl)
